vi "Labeled CRef.vi"   [LabVIEW 2012]
uses:
  CRef Null Address.vi
  XNodes/labelnode/CRef Label Node.xnode
  CRef.lvlib
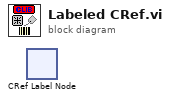
[diagram p0: block diagram]
diagram:
  n1 = xnode "CRef Label Node"() -> ()  [unwired: 3 out]
